vi "Destructor.vi"(8 "error in":errorcluster, 11 "TDMS in":refnum<class "TDMS.lvclass">) -> (0 "error out":errorcluster, 3 "TDMS out":refnum<class "TDMS.lvclass">)   [LabVIEW 2011, in "TDMS.lvclass"]
uses:
  TDMS.lvclass
  TDMS.lvclass/TDMS.ctl
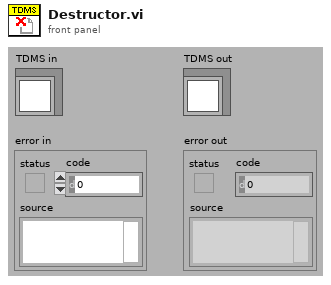
[diagram p1: front panel]
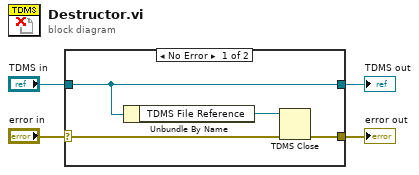
[diagram p0: block diagram]
diagram:
  n1 = case shown="No Error" "error in" {
    selector: "error in" -> [w6 w10]
    tunnel: [w5 w10] -> w3
    tunnel: [w8 w9] -> w1
    tunnel: "TDMS in" -> [w8 w9]
    frame No Error {
      n2 = Unbundle By Name(w8) -> ("TDMS File Reference"=w7:refnum<k34>)
      n3 = TDMS Close(8:w6, 11:w7) -> (0:w5:errorcluster)  [unwired: 1 out]
    }
    frame Error {
    }
  }
  "error out" <- w3
  "TDMS out" <- w1
